vi "UTILITY Save Data.vi"(8 "error in":errorcluster, 10 "Data":string[](array[string]), 11 "refnum":refnum<file>) -> (0 "error out":errorcluster, 3 "refnum out":refnum<file>)   [LabVIEW 2020]
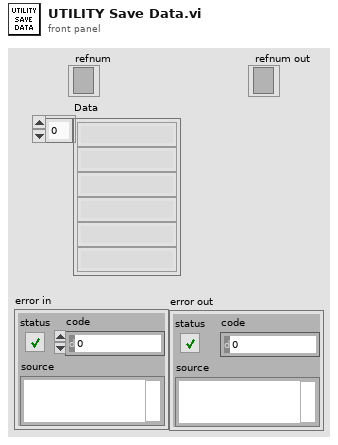
[diagram p1: front panel]
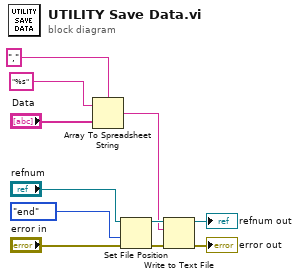
[diagram p0: block diagram]
diagram:
  n1 = Array To Spreadsheet String(delimiter (Tab)=",", array="Data", 3:"%s" ("format string")) -> (spreadsheet string=w6:string)
  n2 = Set File Position(refnum="refnum", from (0:start)=enum16{"start", "end", "current"}."end", error in="error in") -> (refnum out=w9:refnum<file>, error out=w10:errorcluster)  [unwired: 1 in]
  n3 = Write to Text File(file (use dialog)=w9, text=w6, error in=w10) -> (refnum out=→"refnum out":refnum<file>, error out=→"error out":errorcluster)  [unwired: 1 in, 1 out]
